vi "Analog PWM Tester.vi"() -> ()   [LabVIEW 2021]
uses:
  <vilib>/DAQmx/write.llb/DAQmx Write (Analog Wfm 1Chan NSamp).vi
  <vilib>/DAQmx/create/channels.llb/DAQmx Create Channel (AO-Voltage-Basic).vi
  <vilib>/DAQmx/configure/timing.llb/DAQmx Timing (Sample Clock).vi
  <vilib>/DAQmx/miscellaneous.llb/DAQmx Fill In Error Info.vi
  <resource>/objmgr/daqmx.rc
  <vilib>/measure/NI_MABase.lvlib
panel:
  in  "Num Samples":dbl
  in  "sample rate":dbl=1000.0 format="%0.2f"
  in  "STOP":bool
  in  "duty cycle (%)":dbl(slide)=50.0 scale=5.0..10.0
  in  "PWM Control (Analog Out)":tag="myDAQ1/ao1"
  out "PWM Control Signal":waveform(dbl)(graph)={"t0"=timestamp(0 s since 1904-01-01), "dt"=0.001, "Y"=[0.0, 0.0, 0.0, 0.0, 0.0, 0.0, 0.0, 0.0, 0.0, 0.0, 0.0, 0.0, 0.0, 0.0, 0.0, 0.0, 0.0, 0.0, 0.0, 0.0, 0.0, 0.0, 0.0, 0.0, 0.0, 0.0, 0.0, 0.0, 0.0, 0.0, 0.0, 0.0, 0.0, 0.0, 0.0, 0.0, 0.0, 0.0, 0.0, 0.0, 0.0, 0.0, 0.0, 0.0, 0.0, 0.0, 0.0, 0.0, 0.0, 0.0]}
  # "At 50 Hz, 5% DC represents a time on of 1000 us (full reverse)\n                7.5% DC represents a time on of 1500 us (neutral)\n                10% DC represents a time on of 2000 us (full forward)"
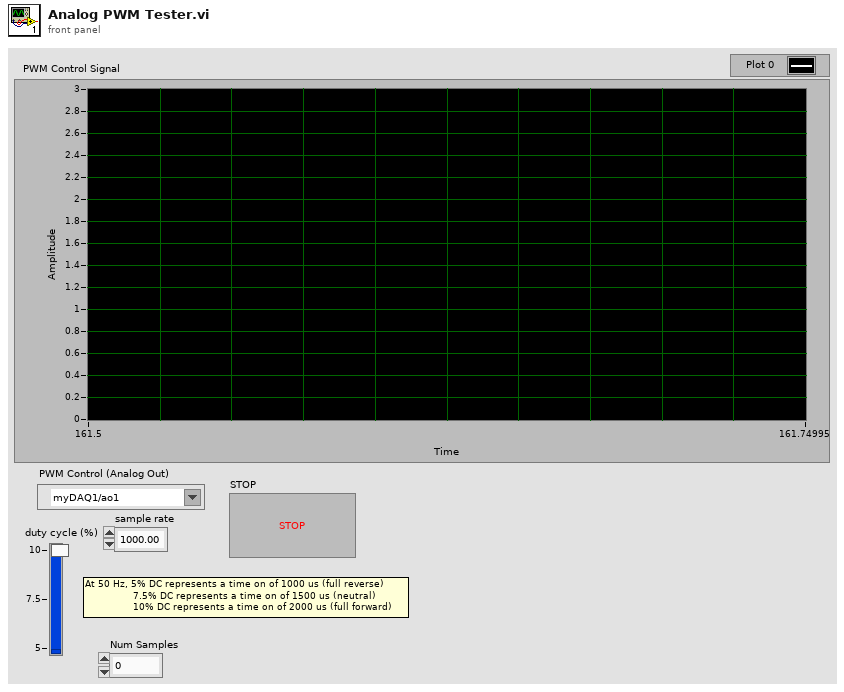
[diagram p1: front panel]
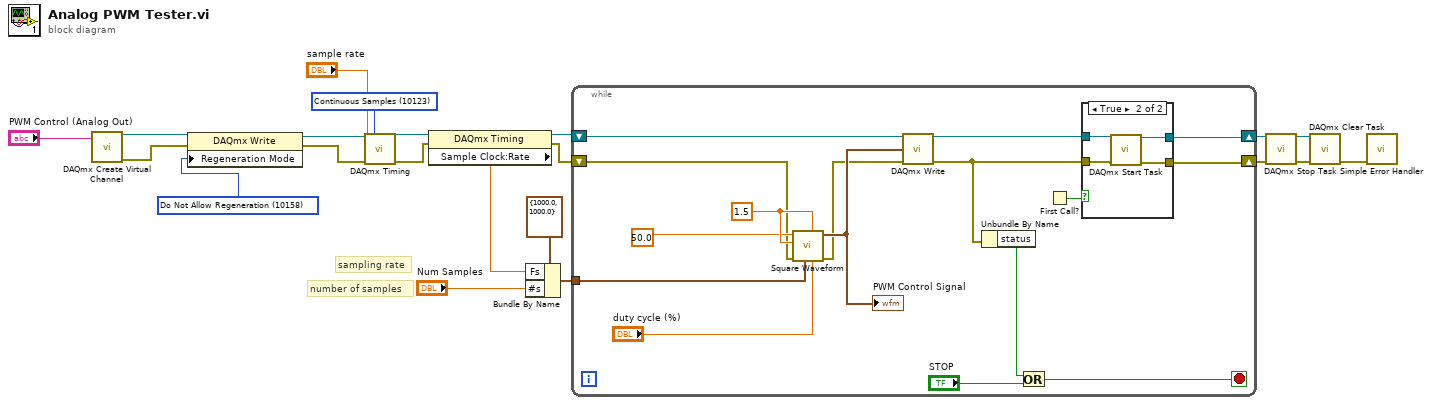
[diagram p0: block diagram]
diagram:
  w10 = 10123 items=["Finite Samples"=10178, "Continuous Samples"=10123, "Hardware Timed Single Point"=12522] ("sample mode")
  w11 = 10158 items=["Allow Regeneration"=10097, "Do Not Allow Regeneration"=10158] ("RegenMode")
  # "number of samples"
  # "sampling rate"
  n1 = call-poly <vilib>:"DAQmx Create Virtual Channel.vi"("physical channels"="PWM Control (Analog Out)") -> ("task out"=w15:refnum<k21>, "error out"=w14:errorcluster)  [unwired: 13 in]
  n2 = property class="DAQmx Write"(reference=w15, error in=w14, "Regeneration Mode"=w11) -> (reference out=w13:refnum<k21>, error out=w12:errorcluster)
  n3 = call-poly <vilib>:"DAQmx Timing.vi"("task/channels in"=w13, "sample mode"=w10, "rate"="sample rate", "error in"=w12) -> ("task out"=w8:refnum<k21>, "error out"=w7:errorcluster)  [unwired: 10 in]
  n4 = property class="DAQmx Timing"(reference=w8, error in=w7) -> (reference out=w5:refnum<k21>, error out=w6:errorcluster, "Sample Clock:Rate"=w2:dbl)
  n5 = Bundle By Name(cluster=cluster{"Fs":dbl, "#s":dbl} {"Fs"=1000.0, "#s"=1000.0} ("sampling info"), "Fs"=w2, "#s"="Num Samples") -> (w3:cluster{"Fs":dbl, "#s":dbl})
  n6 = while {
    shift-right: [w29] -> w17
    shift-left: w5 -> [w37]
    shift-right: [w30] -> w16
    shift-left: w6 -> [w25]
    tunnel: w3 -> [w23]
    stop <- w34 stop-if-true
    w27 = 1.5 ("amplitude")
    n7 = call <vilib>:"Square Waveform.vi"("duty cycle (%)"="duty cycle (%)", "offset"=w27, "sampling info"=w23, "error in (no error)"=w25, "amplitude"=w27, "frequency"=50.0) -> ("error out"=w24:errorcluster, "signal out"=w28:waveform(dbl))  [unwired: 4 in]
    "PWM Control Signal" <- w28
    n8 = call-poly <vilib>:"DAQmx Write.vi"("task/channels in"=w37, "data"=w28, "error in"=w24) -> ("task out"=w32:refnum<k21>, "error out"=w31:errorcluster)  [unwired: 10 in, 1 out]
    n9 = Unbundle By Name(w31) -> ("status"=w36:bool)
    n10 = Or(x=w36, y="STOP") -> (x .or. y?=w34:bool)
    n11 = First Call?() -> (First Call?: T/F=w33:bool)
    n12 = case shown="True" w33 {
      tunnel: w32 -> [w39 w43]
      tunnel: w31 -> [w38 w42]
      tunnel: [w38 w41] -> w30
      tunnel: [w39 w40] -> w29
      frame False {
      }
      frame True {
        n13 = call <vilib>:"DAQmx Start Task.vi"("task/channels in"=w43, "error in"=w42) -> ("task out"=w40:refnum<k21>, "error out"=w41:errorcluster)  [unwired: 12 in]
      }
    }
  }
  n14 = call <vilib>:"DAQmx Stop Task.vi"("task/channels in"=w17, "error in"=w16) -> ("task out"=w21:refnum<k21>, "error out"=w20:errorcluster)  [unwired: 12 in]
  n15 = call <vilib>:"DAQmx Clear Task.vi"("task in"=w21, "error in"=w20) -> ("error out"=w18:errorcluster)  [unwired: 13 in]
  n16 = call <vilib>:"Simple Error Handler.vi"("error in (no error)"=w18) -> ()  [unwired: 4 in, 5 out]
